vi "power PID - V1.vi"(4 "delta time(sec)":dbl=300.0, 6 "nonzero temperature":dbl=300.0, 8 "adaptive sweep settings":T1={"time gap (min) "=0.0, "Bypass error dialog"=TRUE, "range factor"=1.05, "min gamma(kHz)"=0.005, "max step(Hz)"=1.05, "min step(Hz)"=0.005, "save freq units"=enum."Hz", "Zero signal?"=FALSE, "time in Gamma --OK"=FALSE, "scan mode"=enum."predictive", "power control mode "=enum."power vs Temp", "time-in-gamma mode"=enum."same for all"}, 10 "sweep folder path":path, 11 "Fast sweep settings":T4={"Update rate (Hz)"=250.0, "Start F, Hz"=300000.0, "Stop F"=3500000.0, "Number of points"=23000, "Amplitude"=0.2, "Init&amplitude"=TRUE, "IF"=1000.0, "Time constant"=0.001} {"IF" format="%#_6p"; "Amplitude" min=0.0 max=2.5; "Number of points" format="%.0p"; "Stop F" format="%#_6p"; "Start F, Hz" format="%#_6p"; "Update rate (Hz)" format="%0.2f"}) -> (0 "adaptive sweep settings OUT":T1={"time gap (min) "=0.0, "Bypass error dialog"=TRUE, "range factor"=1.05, "min gamma(kHz)"=0.005, "max step(Hz)"=1.05, "min step(Hz)"=0.005, "save freq units"=enum."Hz", "Zero signal?"=FALSE, "time in Gamma --OK"=FALSE, "scan mode"=enum."predictive", "power control mode "=enum."power vs Temp", "time-in-gamma mode"=enum."same for all"}, 1 "frequencies":dbl[](array[numeric]), 2 "temperatures":dbl[](array[numeric]), 3 "Fast sweep settings out":T4={"Update rate (Hz)"=250.0, "Start F, Hz"=200000.0, "Stop F"=1700000.0, "Number of points"=30000, "Amplitude"=2.1, "Init&amplitude"=TRUE, "IF"=1000.0, "Time constant"=0.1} {"IF" format="%#_6p"; "Amplitude" min=0.0 max=2.5; "Number of points" format="%.0p"; "Stop F" format="%#_6p"; "Start F, Hz" format="%#_6p"; "Update rate (Hz)" format="%0.2f"})   [LabVIEW 2016]
uses:
  resonant_ultrasound/Libraries/RUS/Controls/Sweep settings.ctl
  adaptive sweep UI controls.ctl
  next chunk -- algorithm.ctl
  time in gamma mode control.ctl
  ctl -- name dispatcher -- action.ctl
panel:
  out "voltage":dbl
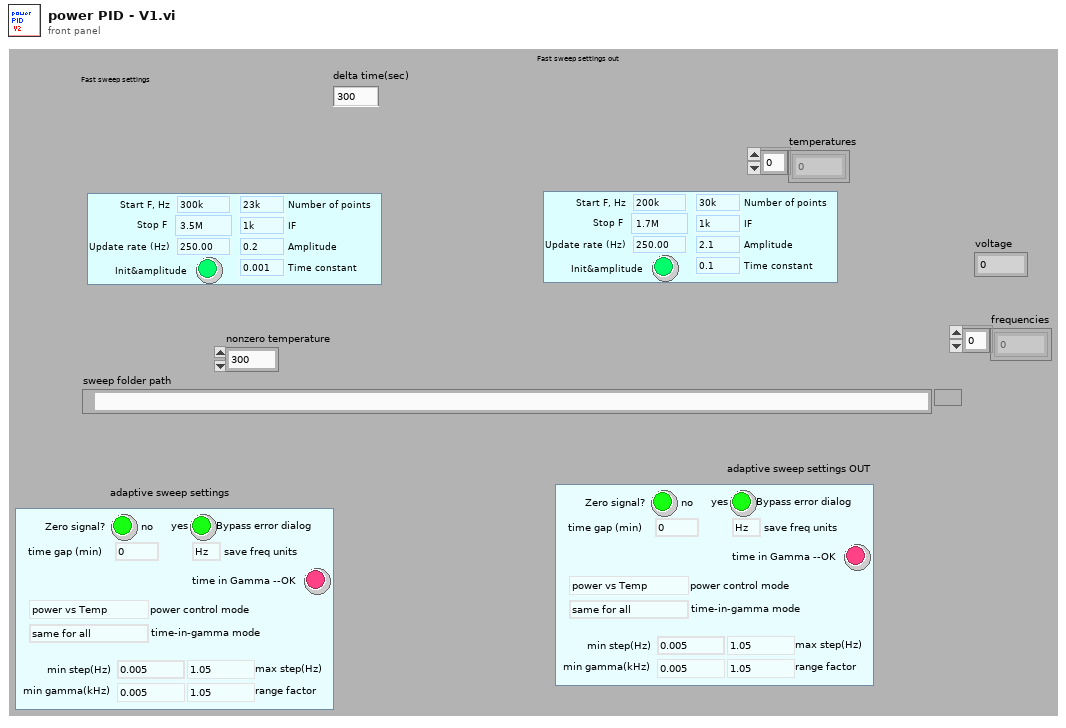
[diagram p1: front panel]
types:
  T1 = typedef "adaptive sweep UI controls.ctl" = cluster{"time gap (min) ":dbl, "Bypass error dialog":bool, "range factor":dbl, "min gamma(kHz)":dbl, "max step(Hz)":dbl, "min step(Hz)":dbl, "save freq units":enum16{"kHz", "Hz"}, "Zero signal?":bool, "time in Gamma --OK":bool, "scan mode":T2, "power control mode ":enum16{"power vs Temp", "power vs Time", "none"}, "time-in-gamma mode":T3}
  T2 = typedef "next chunk -- algorithm.ctl" = enum16{"peak position is known", "uniform", "predictive"}
  T3 = typedef "time in gamma mode control.ctl" = enum16{"same for all", "each one different", "uniform scan"}
  T4 = typedef "Sweep settings.ctl" = cluster{"Update rate (Hz)":dbl, "Start F, Hz":dbl, "Stop F":dbl, "Number of points":i32, "Amplitude":dbl, "Init&amplitude":bool, "IF":dbl, "Time constant":dbl}
  T5 = typedef "ctl -- name dispatcher -- action.ctl" = enum16{"peak frequency", "peak frequency DUMP", "peak gamma DUMP", "peak gamma", "peak frequency TEST", "peak gamma TEST", "ultrasonic power", "time in gamma", "set temperature ", "set temperature timer", "peak default gamma", "last scan file", "peak freq gamma TEST", "peak NAMES", "errors", "P_I_D", "P", "I", "D", "power vs time", "power vs time TIMER", "void", "power log", "set temperature - SINE", "itc ltc log", "peak - time in gamma"}
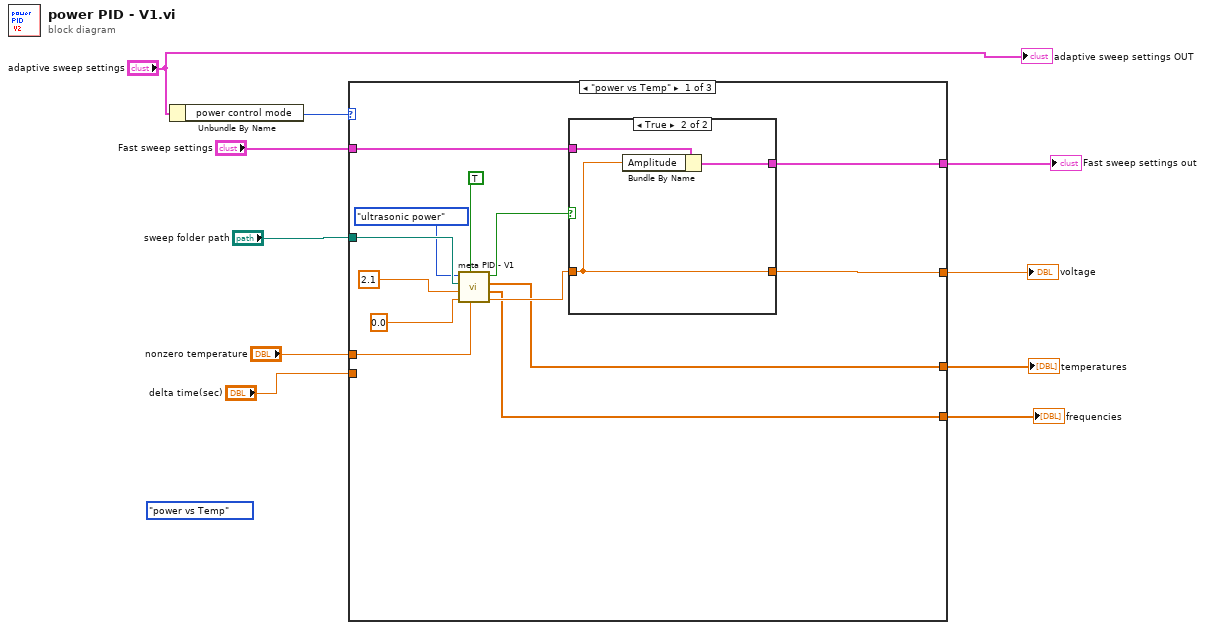
[diagram p0: block diagram]
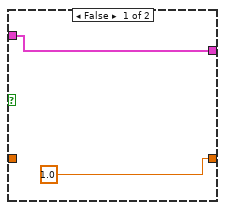
[diagram p2: hidden frame]
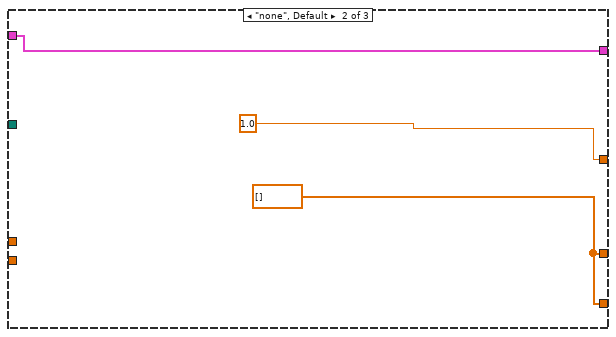
[diagram p3: hidden frame]
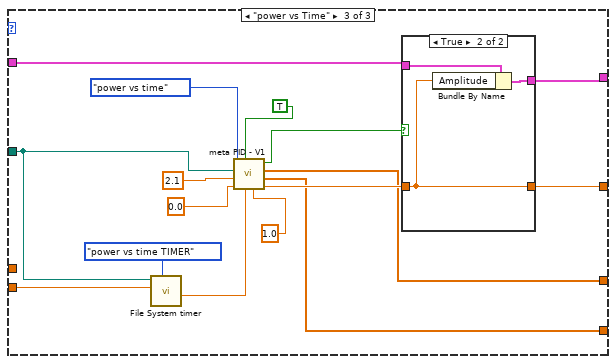
[diagram p4: hidden frame]
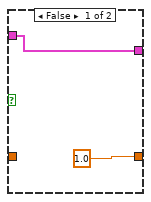
[diagram p5: hidden frame]
diagram:
  (unwired) enum16{"power vs Temp", "power vs Time"}."power vs Temp"
  n1 = Unbundle By Name("adaptive sweep settings") -> ("power control mode"=w1:enum16{"power vs Temp", "power vs Time", "none"})
  n2 = case shown="\"power vs Temp\"" w1 {
    tunnel: [w23 1.0 ("upper") w36] -> w6
    tunnel: "sweep folder path" -> [w20 _ w33]
    tunnel: "nonzero temperature" -> [w19 _ _]
    tunnel: [w17 w29 w37] -> w4
    tunnel: [w16 w29 w38] -> w5
    tunnel: "Fast sweep settings" -> [w15 w30 w41]
    tunnel: [w13 w30 w39] -> w7
    tunnel: "delta time(sec)" -> [_ _ w47]
    frame "power vs Temp" {
      n3 = call "meta PID - V1.vi"("input parameter"=w19, "control?"=TRUE, "lower limit"=0.0 ("lower"), "upper limit"=2.1 ("upper"), "sweep folder path"=w20, "ctl name dispatch"=ctl_--_name_dispatcher_--_action."ultrasonic power") -> ("bezier output"=w18:dbl, "frequencies"=w17:dbl[], "temperatures"=w16:dbl[], "ok"=w14:bool)  [unwired: 2 in]
      n4 = case shown="True" w14 {
        tunnel: [w24 w28] -> w13
        tunnel: [1.0 ("upper") w27] -> w23
        tunnel: w18 -> [_ w27]
        tunnel: w15 -> [w24 w26]
        frame False {
        }
        frame True {
          n5 = Bundle By Name(cluster=w26, "Amplitude"=w27) -> (w28:T4)
        }
      }
    }
    frame "none", Default {
      w29 = dbl[] [] ("temperatures")
    }
    frame "power vs Time" {
      n6 = call "File System timer.vi"("ctl kind IN 2"=ctl_--_name_dispatcher_--_action."power vs time TIMER" ("ctl kind IN"), "delta time(sec)"=w47, "sweep folder path"=w33) -> ("time (min)"=w43:dbl)  [unwired: 8 in]
      n7 = call "meta PID - V1.vi"("default output"=1.0 ("upper"), "input parameter"=w43, "control?"=TRUE, "lower limit"=0.0 ("lower"), "upper limit"=2.1 ("upper"), "sweep folder path"=w33, "ctl name dispatch"=ctl_--_name_dispatcher_--_action."power vs time") -> ("bezier output"=w40:dbl, "frequencies"=w37:dbl[], "temperatures"=w38:dbl[], "ok"=w42:bool)  [unwired: 1 in]
      n8 = case shown="True" w42 {
        tunnel: [w48 w52] -> w39
        tunnel: [1.0 ("upper") w51] -> w36
        tunnel: w40 -> [_ w51]
        tunnel: w41 -> [w48 w50]
        frame False {
        }
        frame True {
          n9 = Bundle By Name(cluster=w50, "Amplitude"=w51) -> (w52:T4)
        }
      }
    }
  }
  "Fast sweep settings out" <- w7
  "voltage" <- w6
  "temperatures" <- w5
  "frequencies" <- w4
  "adaptive sweep settings OUT" <- "adaptive sweep settings"
